vi "BusClassTestBed.vi"() -> ()   [LabVIEW 2017, in "Bus_class.lvlib" / "Bus.lvclass"]
uses:
  Bus.lvclass
  Public/TypeDefs/clBusData.ctl
  FrontPanel/TypeDefs/clEventConfig.ctl
  Modules/PmuImpairPlugins/PmuImpairPluginBase_class/TypeDefs/clImpairConfig.ctl
  Modules/EventPlugins/EventPluginBaseClass/TypeDefs/clEvtReportArray.ctl
  Modules/EventPlugins/EventPluginBaseClass/TypeDefs/clEvtReport.ctl
  Modules/EventPlugins/EventPluginBaseClass/TypeDefs/dblEvtSignalArray.ctl
  Modules/NetworkImpairmentModule/PublicAPI/Arguments/Broadcasts/dblNetworkTime.ctl
  Modules/NetworkImpairmentModule/PublicAPI/Arguments/Broadcasts/dblPktLoss.ctl
  Modules/FlagImpairModule/PublicAPI/Arguments/Broadcasts/ui32FlagImpairmentArray.ctl
  Modules/OutputToFilePlugins/OutputToFileBasePlugin/Typedefs/PmuCfgOpt.ctl
  FrontPanel/TypeDefs/clFrontPanelControlRefs.ctl
  Modules/EventModule/PublicAPI/Arguments/Broadcasts/clStatUpdate.ctl
  Framework.lvlib
  <userlib>/NIST/NISTErrorLib/NISTErrorLib.lvlib
  Modules/EventModule/EventModule.lvlib
  Modules/PmuImpairModule/PmuImpairModule.lvlib
  Modules/NetworkImpairmentModule/NetworkImpairmentModule.lvlib
  Modules/FlagImpairModule/FlagImpairModule.lvlib
  Modules/OutputToFileModule/OutputToFileModule.lvlib
  Modules/EventPlugins/EventPluginBaseClass/EventPluginBaseClass.lvclass
  Modules/OutputToFilePlugins/OutputToFileBasePlugin/OutputToFileBasePlugin.lvclass
  Modules/PmuImpairPlugins/PmuImpairPluginBase_class/PmuImpairPluginBase.lvclass
panel:
  in  "Network Impairment Type":u16(ring) items=["Network Impairment"]
  in  "btnTestScript":bool
  in  "Script":string[](array[string])=["GetEvtReports", "GetEvtSignal", "TransferEvtReportsToPmuImpair", "TransferEvtSignalToPmuImpair", "GetPmuRepairReports", "Stop"]
  in  "Flag Impairment Type":u16(ring) items=["C37.118", "IEC61850"]
  in  "Test File":string
  in  "PMU Impairment Type":u16(ring) items=["C37.118.1 Model", "Sine Model", "UserPmuImpair1"]
  in  "Event Type":u16(ring) items=["C37.118.1", "Frequency Ramp", "Modulation", "Steady State", "Step", "User1", "User2"]
  in  "clBusData":T1={"BusNumber"=0, "EvtPluginINIFilePath"=path "", "EvtParams"=[], "EvtConfig"={"UTC Time 0"=timestamp(0 s since 1904-01-01), "Nominal Frequency"=60, "Reporting Rate"=60, "Fsamp"=960, "PosSeq"=FALSE}, "Start Time"=0.0, "End Time"=0.0, "PmuImpairPluginINIFilePath"=path "", "PmuImpairParams "=[["8.19"], ["164"]], "PmuImpairConfig"={"FilterType"="Hamming", "bPosSeq"=TRUE}, "NetImpPluginINIFilePath"=path "", "NetImpParams"=[], "FlagImpPluginINIFilePath"=path "", "FlagImpParams"=[], "EvtReportArray"=[], "EventSignalArray"=[], "ImpairReportArray"=[], "NetworkTime"=[], "PktLoss"=[], "FlagImpArray"=[], "OutputToFilePluginINIFilePath"=path "", "Output File Path"=path "", "clConfigOptions"={"TIME_BASE"=1000000, "STN"="Bus_1", "IDCODE"=0, "rdoPolRect"=enum."Rectangular", "rdoFloatInt"=enum."Float", "PHUNIT"=1000000, "rdoFreqDfreq"=enum."Float", "CHNAM"=["VA", "VB", "VC", "V+", "IA", "IB", "IC", "I+"], "chkCfg2Prefix"=TRUE}, "AppPluginINIFilePath"=path "", "AppConfig"=variant, "AppOutput"=variant} {"clConfigOptions"."PHUNIT" max=16777216 step=1 format="%08d"; "clConfigOptions"."IDCODE" format="%02x"; "clConfigOptions"."TIME_BASE" max=16777216 step=1 format="%08d"; "ImpairReportArray"."Synx" format="%#_4g"; "EvtReportArray"."Synx" format="%#_4g"; "EvtConfig"."Reporting Rate" items=["10 FPS"=10, "12 FPS"=12, "15 FPS"=15, "20 FPS"=20, "25 FPS"=25, "30 FPS"=30, "50 FPS"=50, "60 FPS"=60]; "EvtConfig"."Nominal Frequency" items=["50 Hz"=50, "60 Hz"=60]}
  in  "btnExit":bool
  in  "btnRemoveBus":bool
  in  "btnAddBus":bool
  out "Number of Buses":u8 min=1
  in  "Bus Number":u8(ring) items=["", "1"]
  out "Status Log":string
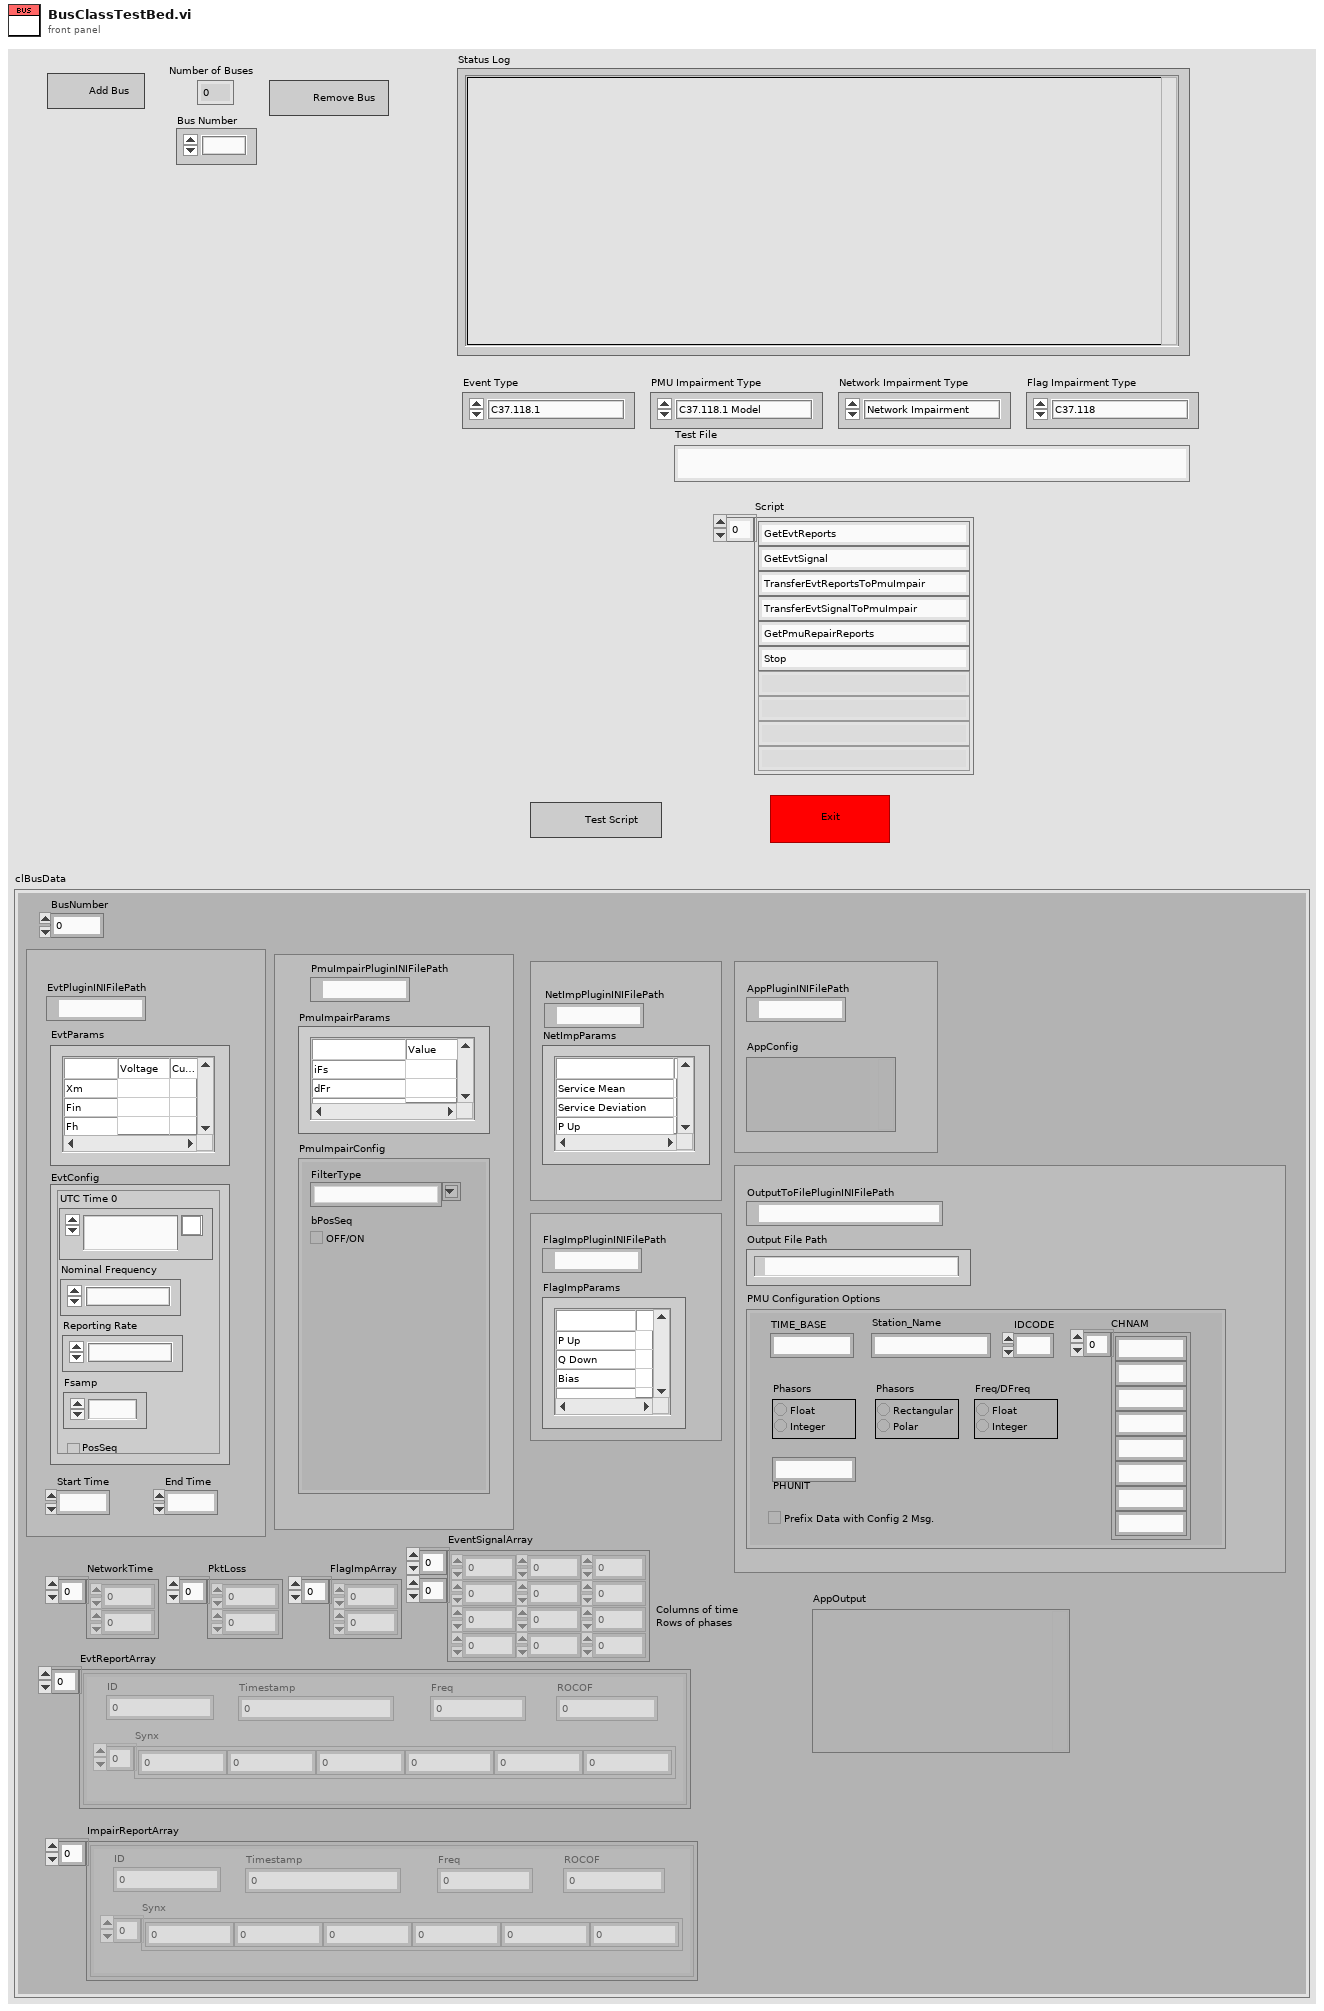
[diagram p1: front panel]
types:
  T1 = typedef "Bus_class.lvlib/Bus.lvclass/clBusData.ctl" = cluster{"BusNumber":u8, "EvtPluginINIFilePath":path, "EvtParams":string[][], "EvtConfig":T2, "Start Time":dbl, "End Time":dbl, "PmuImpairPluginINIFilePath":path, "PmuImpairParams ":string[][], "PmuImpairConfig":T3, "NetImpPluginINIFilePath":path, "NetImpParams":string[][], "FlagImpPluginINIFilePath":path, "FlagImpParams":string[][], "EvtReportArray":T4, "EventSignalArray":T6, "ImpairReportArray":T4, "NetworkTime":T7, "PktLoss":T8, "FlagImpArray":T9, "OutputToFilePluginINIFilePath":path, "Output File Path":path, "clConfigOptions":T10, "AppPluginINIFilePath":path, "AppConfig":variant, "AppOutput":variant}
  T2 = typedef "Framework.lvlib/clEventConfig.ctl" = cluster{"UTC Time 0":timestamp, "Nominal Frequency":u16, "Reporting Rate":u16, "Fsamp":u32, "PosSeq":bool}
  T3 = typedef "PmuImpairPlugins.lvlib/PmuImpairPluginBase.lvclass/clImpairConfig.ctl" = cluster{"FilterType":string, "bPosSeq":bool}
  T4 = typedef "EventPlugins.lvlib/EventPluginBaseClass.lvclass/clEvtReportArray.ctl" = T5[]
  T5 = typedef "EventPlugins.lvlib/EventPluginBaseClass.lvclass/clEvtReport.ctl" = cluster{"Timestamp":dbl, "Synx":cdb[], "Freq":dbl, "ROCOF":dbl, "ID":i16}
  T6 = typedef "EventPlugins.lvlib/EventPluginBaseClass.lvclass/dblEvtSignalArray.ctl" = dbl[][]
  T7 = typedef "NetworkImpairmentModule.lvlib/dblNetworkTime.ctl" = dbl[]
  T8 = typedef "NetworkImpairmentModule.lvlib/dblPktLoss.ctl" = dbl[]
  T9 = typedef "FlagImpairModule.lvlib/ui32FlagImpairmentArray.ctl" = u32[]
  T10 = typedef "OutputToFilePlugins.lvlib/OutputToFileBasePlugin.lvclass/PmuCfgOpt.ctl" = cluster{"TIME_BASE":u64, "STN":string, "IDCODE":u16, "rdoPolRect":enum32{"Rectangular", "Polar"}, "rdoFloatInt":enum32{"Float", "Integer"}, "PHUNIT":u64, "rdoFreqDfreq":enum32{"Float", "Integer"}, "CHNAM":string[], "chkCfg2Prefix":bool}
  T11 = typedef "Framework.lvlib/clFrontPanelControlRefs.ctl" = cluster{"TestFilePathRef":refnum<vi>, "BusNumberRef":refnum<vi>, "NumberOfBusesRef":refnum<vi>, "EvtTypeRef":refnum<vi>, "EvtParamsRef":refnum<vi>, "EvtConfigRef":refnum<vi>, "StartTimeRef":refnum<vi>, "EndTimeRef":refnum<vi>, "PmuImpairTypeRef":refnum<vi>, "PmuImpairParamsRef":refnum<vi>, "NetImpairParamsRef":refnum<vi>, "FlagImpairTypeRef":refnum<vi>, "FlagImpairParamsRef":refnum<vi>, "NetImpairTypeRef":refnum<vi>, "OutputFileType":refnum<vi>, "PmuImpairConfigRef":refnum<vi>, "AppTypeRef":refnum<vi>, "ScriptPathRef":refnum<vi>, "ShowPanels?":refnum<vi>}
  T12 = typedef "EventModule.lvlib/clBroadcastEvents.ctl" = cluster{"DidInit":refnum<user-event>, "StatusUpdate":refnum<user-event>, "ErrorReport":refnum<user-event>, "DidStop":refnum<user-event>, "ReadEvtConfig":refnum<user-event>, "ReadTimeArray":refnum<user-event>, "ReadEvtParams":refnum<user-event>, "GetEvtReportArray":refnum<user-event>, "ReadPathToPlugin":refnum<user-event>, "GetEvtSignal":refnum<user-event>, "ReadBusNumber":refnum<user-event>}
  T13 = typedef "PmuImpairModule.lvlib/clBroadcastEvents.ctl" = cluster{"DidInit":refnum<user-event>, "StatusUpdate":refnum<user-event>, "ErrorReport":refnum<user-event>, "DidStop":refnum<user-event>, "ImpairConfig":refnum<user-event>, "ImpairParams":refnum<user-event>, "ImpairReports":refnum<user-event>, "PathToPlugin":refnum<user-event>, "BusNumber":refnum<user-event>}
  T14 = typedef "NetworkImpairmentModule.lvlib/clBroadcastEvents.ctl" = cluster{"DidInit":refnum<user-event>, "StatusUpdate":refnum<user-event>, "ErrorReport":refnum<user-event>, "DidStop":refnum<user-event>, "ReadNetImpParams":refnum<user-event>, "ReadLossThreshold":refnum<user-event>, "GetNetworkTime":refnum<user-event>, "GetPktLoss":refnum<user-event>, "ReadPathToPlugin":refnum<user-event>}
  T15 = typedef "FlagImpairModule.lvlib/clBroadcastEvents.ctl" = cluster{"DidInit":refnum<user-event>, "StatusUpdate":refnum<user-event>, "ErrorReport":refnum<user-event>, "DidStop":refnum<user-event>, "ReadFlagImpairConfig":refnum<user-event>, "ReadPluginINIFilePath":refnum<user-event>, "ReadFlagImpairParams":refnum<user-event>, "ReadTimeArray":refnum<user-event>, "GetFlagImpairment":refnum<user-event>}
  T16 = typedef "Framework.lvlib/clRequestEvents.ctl" = cluster{"StopRequest":refnum<user-event>}
  T17 = typedef "OutputToFileModule.lvlib/clBroadcastEvents.ctl" = cluster{"DidInit":refnum<user-event>, "StatusUpdate":refnum<user-event>, "ErrorReport":refnum<user-event>, "DidStop":refnum<user-event>, "PathToPlugin":refnum<user-event>, "PmuConfig":refnum<user-event>, "OutputPath":refnum<user-event>}
  T18 = typedef "EventModule.lvlib/clStatUpdate.ctl" = cluster{"Status":string}
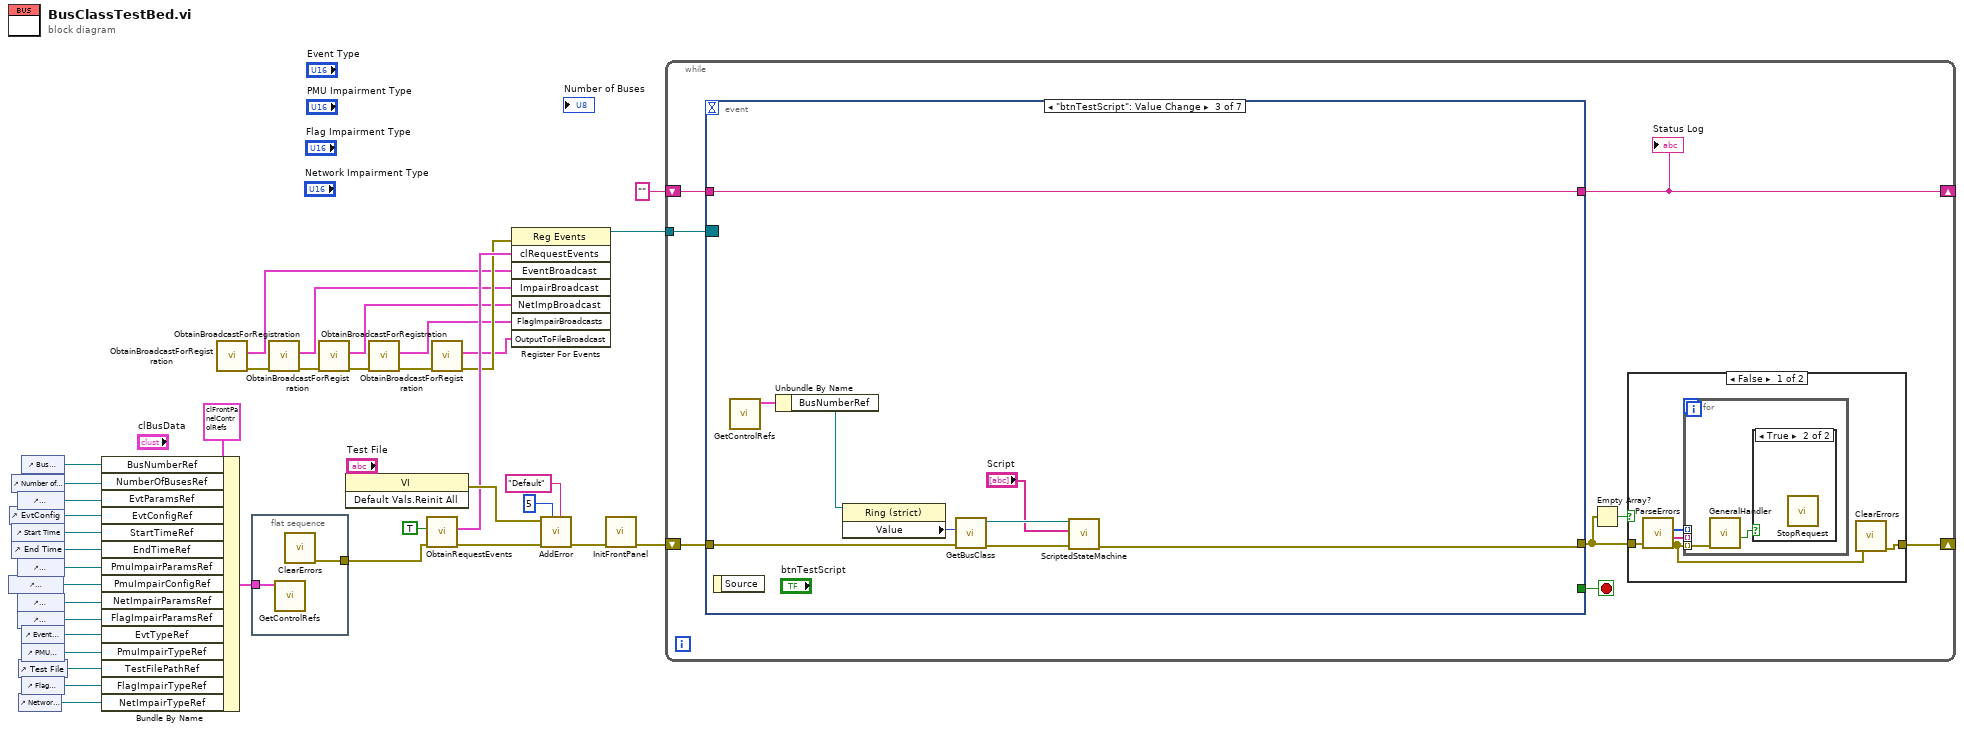
[diagram p0: block diagram]
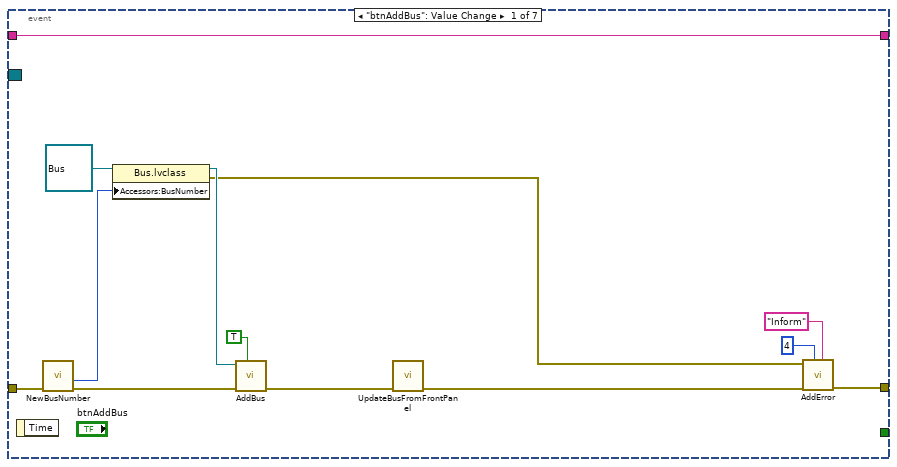
[diagram p4: hidden frame]
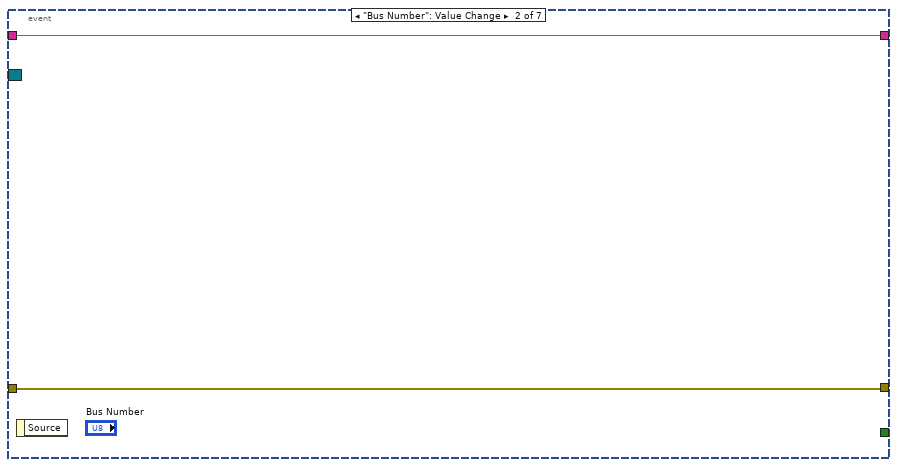
[diagram p5: hidden frame]
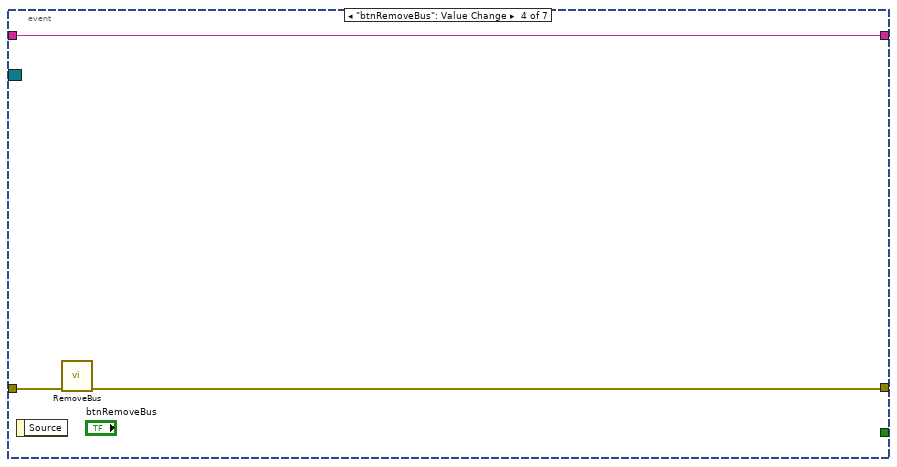
[diagram p6: hidden frame]
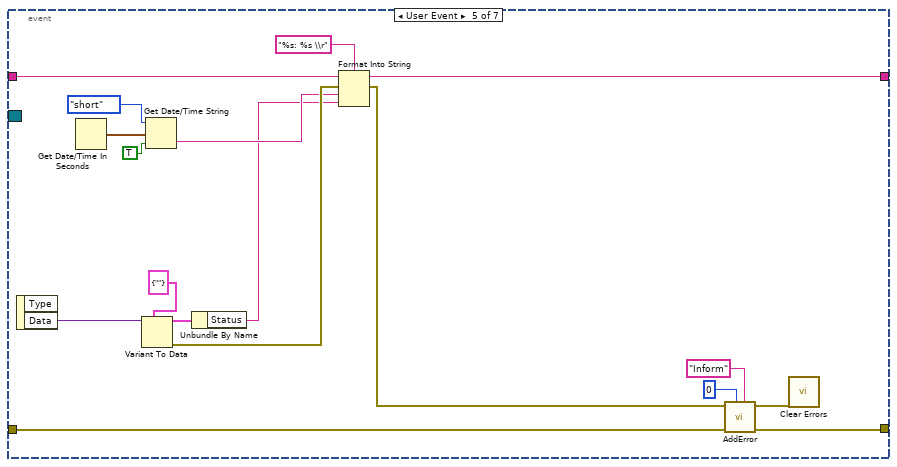
[diagram p7: hidden frame]
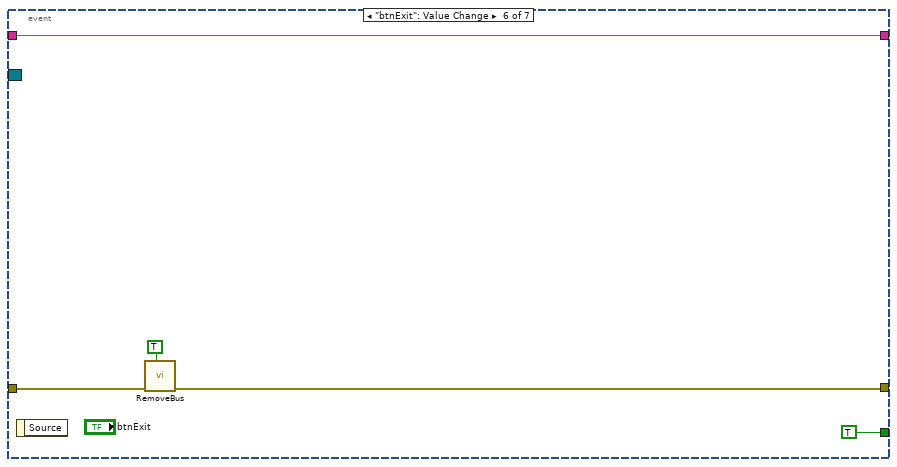
[diagram p8: hidden frame]
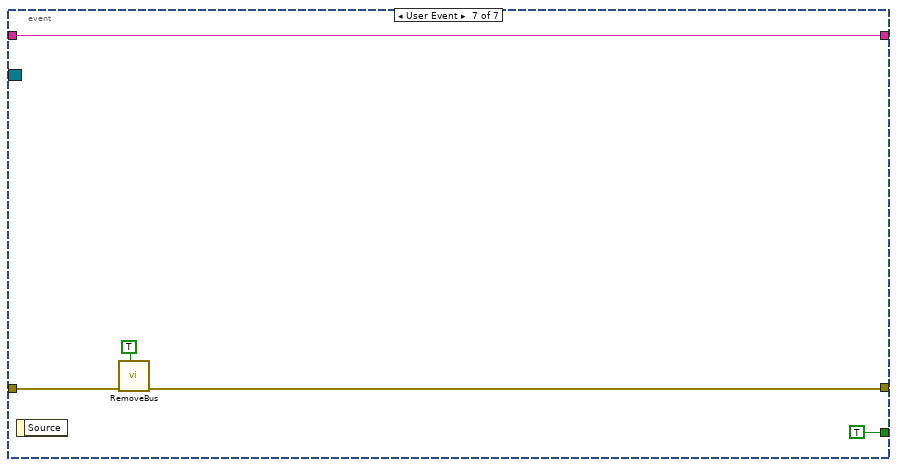
[diagram p9: hidden frame]
diagram:
  n1 = control-ref of="PmuImpairConfig"() -> (w3:refnum<vi>)
  n2 = control-ref of="EvtConfig"() -> (w23:refnum<vi>)
  n3 = control-ref of="Number of Buses"() -> (w36:refnum<vi>)
  n4 = control-ref of="Start Time"() -> (w22:refnum<vi>)
  n5 = control-ref of="End Time"() -> (w21:refnum<vi>)
  n6 = control-ref of="EvtParams"() -> (w24:refnum<vi>)
  n7 = control-ref of="PmuImpairParams"() -> (w20:refnum<vi>)
  n8 = control-ref of="NetImpParams"() -> (w19:refnum<vi>)
  n9 = control-ref of="FlagImpParams"() -> (w18:refnum<vi>)
  n10 = control-ref of="Test File"() -> (w13:refnum<vi>)
  n11 = control-ref of="Network Impairment Type"() -> (w11:refnum<vi>)
  n12 = control-ref of="Bus Number"() -> (w25:refnum<vi>)
  n13 = control-ref of="Event Type"() -> (w17:refnum<vi>)
  n14 = control-ref of="PMU Impairment Type"() -> (w16:refnum<vi>)
  n15 = control-ref of="Flag Impairment Type"() -> (w12:refnum<vi>)
  n16 = Bundle By Name(cluster=T11 {"TestFilePathRef"=refnum, "BusNumberRef"=refnum, "NumberOfBusesRef"=refnum, "EvtTypeRef"=refnum, "EvtParamsRef"=refnum, "EvtConfigRef"=refnum, "StartTimeRef"=refnum, "EndTimeRef"=refnum, "PmuImpairTypeRef"=refnum, "PmuImpairParamsRef"=refnum, "NetImpairParamsRef"=refnum, "FlagImpairTypeRef"=refnum, "FlagImpairParamsRef"=refnum, "NetImpairTypeRef"=refnum, "OutputFileType"=refnum, "PmuImpairConfigRef"=refnum, "AppTypeRef"=refnum, "ScriptPathRef"=refnum, "ShowPanels?"=refnum} ("clFrontPanelControlRefs"), "BusNumberRef"=w25, "NumberOfBusesRef"=w36, "EvtParamsRef"=w24, "EvtConfigRef"=w23, "StartTimeRef"=w22, "EndTimeRef"=w21, "PmuImpairParamsRef"=w20, "PmuImpairConfigRef"=w3, "NetImpairParamsRef"=w19, "FlagImpairParamsRef"=w18, "EvtTypeRef"=w17, "PmuImpairTypeRef"=w16, "TestFilePathRef"=w13, "FlagImpairTypeRef"=w12, "NetImpairTypeRef"=w11) -> (w2:T11)
  n17 = call "ObtainBroadcastForRegistration.vi"() -> ("error out"=w32:errorcluster, "EventBroadcast"=w8:T12)  [unwired: 10 in]
  n18 = flat-sequence {
    tunnel: w2 -> [w40]
    tunnel: [w39] -> w1
    frame #0 {
      n19 = call "GetControlRefs.vi"("clControlRefs In"=w40) -> ()  [unwired: 10 in, 1 out]
      n20 = call <userlib>:"ClearErrors.vi"() -> ("ErrorArray"=w39:errorcluster[])  [unwired: 11 in]
    }
  }
  n21 = call "ObtainBroadcastForRegistration.vi"("error in (no error)"=w32) -> ("error out"=w31:errorcluster, "ImpairBroadcast"=w7:T13)  [unwired: 9 in]
  n22 = call "ObtainBroadcastForRegistration.vi"("error in (no error)"=w31) -> ("error out"=w30:errorcluster, "NetImpBroadcast"=w6:T14)  [unwired: 9 in]
  n23 = invoke class="VI" method="Default Vals.Reinit All"() -> (error out=w35:errorcluster)  [unwired: 3 in, 2 out]
  n24 = call "ObtainBroadcastForRegistration.vi"("error in (no error)"=w30) -> ("error out"=w10:errorcluster, "FlagImpairBroadcasts"=w5:T15)  [unwired: 9 in]
  n25 = call "ObtainRequestEvents.vi"("ErrorArray In"=w1, "CreateNew (F)"=TRUE) -> ("ErrorArray Out"=w28:errorcluster[], "clRequestEvents"=w26:T16)  [unwired: 8 in]
  n26 = call "ObtainBroadcastForRegistration.vi"("error in (no error)"=w10) -> ("error out"=w9:errorcluster, "OutputToFileBroadcast"=w4:T17)  [unwired: 9 in]
  n27 = register-events(error in=w9, w26, w8, w7, w6, w5, w4) -> (reference out=w29:refnum<event-registration>)  [unwired: 1 in, 1 out]
  n28 = call <userlib>:"AddError.vi"("Severity"="Default" ("String"), "Priority"=u8 5, "ErrorArray"=w28, "error in (no error)"=w35) -> ("ErrorArray"=w15:errorcluster[])  [unwired: 6 in, 1 out]
  n29 = call "InitFrontPanel.vi"("ErrorArray In"=w15) -> ("ErrorArray Out"=w14:errorcluster[])  [unwired: 10 in]
  n30 = while {
    shift-right: [w42] -> _
    shift-left: "" ("Status Log") -> [w48]
    shift-right: [w43] -> _
    shift-left: w14 -> [w47]
    tunnel: w29 -> [w46]
    stop <- w41 stop-if-true
    n31 = event shown="[2] \"btnTestScript\": Value Change" {
      selector: w46 -> [_ _ _ _ _ _ _]
      dyn-events: _ -> [_ _ _ _ _ _ _]
      timeout: _ -> [_ _ _ _ _ _ _]
      tunnel: w48 -> [w69 w70 w75 w81 w89 w105 w111]
      tunnel: [w69 w70 w75 w81 w88 w105 w111] -> w42
      tunnel: w47 -> [w68 w71 w80 w83 w94 w104 w109]
      tunnel: [w63 w71 w76 w82 w95 w103 w108] -> w45
      tunnel: [_ _ _ _ _ TRUE TRUE] -> w41
      event "btnAddBus": Value Change {
        n32 = event-data() -> ()  [unwired: 1 in, 1 out]
        n33 = call "NewBusNumber.vi"("ErrorArray In"=w68) -> ("ErrorArray Out"=w65:errorcluster[], "BusNumber"=w66:u8)  [unwired: 9 in]
        n34 = property class="Bus.lvclass"(reference=refnum<class "Bus.lvclass"> refnum ("Framework.lvlib:Bus.lvclass"), "Accessors:BusNumber"=w66) -> (reference out=w64:refnum<class "Bus.lvclass">, error out=w61:errorcluster)  [unwired: 1 in]
        n35 = call "AddBus.vi"("ShowPanels?"=TRUE, "ErrorArray In"=w65, "BusClass In"=w64) -> ("ErrorArray Out"=w59:errorcluster[])  [unwired: 6 in, 2 out]
        n36 = call "UpdateBusFromFrontPanel.vi"("ErrorArray In"=w59) -> ("ErrorArray Out"=w58:errorcluster[])  [unwired: 8 in, 2 out]
        n37 = call <userlib>:"AddError.vi"("Severity"="Inform" ("String"), "Priority"=u8 4, "ErrorArray"=w58, "error in (no error)"=w61) -> ("ErrorArray"=w63:errorcluster[])  [unwired: 6 in, 1 out]
      }
      event "Bus Number": Value Change {
        n38 = event-data() -> ()  [unwired: 1 in, 1 out]
      }
      event "btnTestScript": Value Change {
        n39 = event-data() -> ()  [unwired: 1 in, 1 out]
        n40 = call "GetControlRefs.vi"() -> ("clControlRefs Out"=w72:T11)  [unwired: 11 in]
        n41 = Unbundle By Name(w72) -> ("BusNumberRef"=w74:refnum<vi>)
        n42 = property class="Ring (strict)"(reference=w74) -> ("Value"=w73:u8)  [unwired: 1 in, 2 out]
        n43 = call "GetBusClass.vi"("ErrorArray In"=w80, "BusNumber"=w73) -> ("ErrorArray Out"=w79:errorcluster[], "Framework.lvlib:Bus.lvclass"=w78:refnum<class "Bus.lvclass">)  [unwired: 8 in]
        n44 = call "ScriptedStateMachine.vi"("ErrorArray In"=w79, "Script"="Script", "Bus"=w78) -> ("ErrorArray Out"=w76:errorcluster[])  [unwired: 6 in, 2 out]
      }
      event "btnRemoveBus": Value Change {
        n45 = event-data() -> ()  [unwired: 1 in, 1 out]
        n46 = call "RemoveBus.vi"("ErrorArray In"=w83) -> ("ErrorArray Out"=w82:errorcluster[])  [unwired: 10 in]
      }
      event User Event {
        n47 = event-data() -> ("Data"=w85:variant)  [unwired: 1 in, 1 out]
        n48 = Get Date/Time In Seconds() -> (seconds since 1Jan1904=w99:timestamp)
        n49 = Variant To Data(type=T18 {"Status"=""} ("clStatUpdate"), Variant=w85) -> (data=w92:T18, error out=w98:errorcluster)  [unwired: 1 in]
        n50 = Get Date/Time String(date format (0)=enum16{"short", "long", "abbreviated"}."short", seconds (now)=w99, want seconds? (F)=TRUE) -> (time string=w97:string)  [unwired: 1 out]
        n51 = Unbundle By Name(w92) -> ("Status"=w84:string)
        n52 = Format Into String(format string="%s: %s \\r", initial string=w89, error in=w98, w97, w84) -> (resulting string=w88:string, error out=w93:errorcluster)
        n53 = call <userlib>:"AddError.vi"("Severity"="Inform" ("String"), "Priority"=u8 0, "ErrorArray"=w94, "error in (no error)"=w93) -> ("ErrorArray"=w95:errorcluster[], "error out"=w87:errorcluster)  [unwired: 6 in]
        n54 = call <vilib>:"Clear Errors.vi"("error in (no error)"=w87) -> ()  [unwired: 5 in, 2 out]
      }
      event "btnExit": Value Change {
        n55 = event-data() -> ()  [unwired: 1 in, 1 out]
        n56 = call "RemoveBus.vi"("Remove All? (F)"=TRUE, "ErrorArray In"=w104) -> ("ErrorArray Out"=w103:errorcluster[])  [unwired: 9 in]
      }
      event User Event {
        n57 = event-data() -> ()  [unwired: 1 in, 1 out]
        n58 = call "RemoveBus.vi"("Remove All? (F)"=TRUE, "ErrorArray In"=w109) -> ("ErrorArray Out"=w108:errorcluster[])  [unwired: 9 in]
      }
    }
    "Status Log" <- w42
    n59 = Empty Array?(array=w45) -> (empty?=w44:bool)
    n60 = case shown="False" w44 {
      tunnel: w45 -> [w53 w56]
      tunnel: [w49 w56] -> w43
      frame False {
        n61 = call <userlib>:"ParseErrors.vi"("ErrorArray"=w53) -> ("ErrorArray"=w50:errorcluster[], "Severity"=w52:string[], "Priority"=w51:i32[])  [unwired: 8 in]
        n62 = for {
          tunnel: w50 -> [w55] mode=indexing
          tunnel: w52 -> [_] mode=indexing
          tunnel: w51 -> [_] mode=indexing
          n63 = call <userlib>:"GeneralHandler.vi"("error in (no error)"=w55) -> ("Stop"=w54:bool)  [unwired: 7 in, 3 out]
          n64 = case shown="True" w54 {
            frame False {
            }
            frame True {
              n65 = call "StopRequest.vi"() -> ()  [unwired: 11 in, 1 out]
            }
          }
        }
        n66 = call <userlib>:"ClearErrors.vi"("ErrorArray"=w50) -> ("ErrorArray"=w49:errorcluster[])  [unwired: 10 in]
      }
      frame True {
      }
    }
  }
